vi "KMCS2000 Steps.vi"(9 "Step 1":dbl, 10 "Start (V)":dbl, 11 "Mid (V)":dbl) -> (2 "Step sizeand direction":dbl, 3 "Number of steps":dbl)   [LabVIEW 2018]
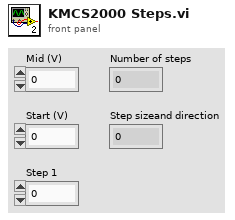
[diagram p1: front panel]
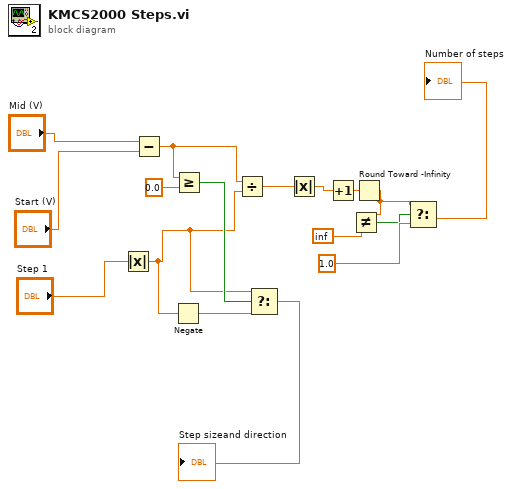
[diagram p0: block diagram]
diagram:
  n1 = Absolute Value(x="Step 1") -> (abs(x)=w11:dbl)
  n2 = Subtract(x="Mid (V)", y="Start (V)") -> (x-y=w14:dbl)
  n3 = Negate(x=w11) -> (-x=w12:dbl)
  n4 = Greater Or Equal?(x=w14, y=0.0) -> (x >= y?=w15:bool)
  n5 = Divide(x=w14, y=w11) -> (x/y=w3:dbl)
  n6 = Select(t=w11, s=w15, f=w12) -> (s? t:f=→"Step sizeand direction":dbl)
  n7 = Absolute Value(x=w3) -> (abs(x)=w4:dbl)
  n8 = Increment(x=w4) -> (x+1=w5:dbl)
  n9 = Round Toward -Infinity(1:w5) -> (0:w8:dbl)
  n10 = Not Equal?(x=w8, y=inf) -> (x != y?=w7:bool)
  n11 = Select(t=w8, s=w7, f=1.0) -> (s? t:f=→"Number of steps":dbl)
